vi "Status Monitor (Multi Unit).vi"() -> ()   [LabVIEW 2017, in "Status Monitor Library.lvlib"]
uses:
  Status Monitor Library.lvlib
  Communications/Typedefs/DTACQ Module Carrier Status.ctl
  Communications/Typedefs/DTACQ Status--Enum.ctl
  Communications/Communications Library.lvlib
panel:
  in  "error out":errorcluster
  out "Array":T1[](array[typedef])
  in  "stop":bool
  in  "appended array":path[](array[path])
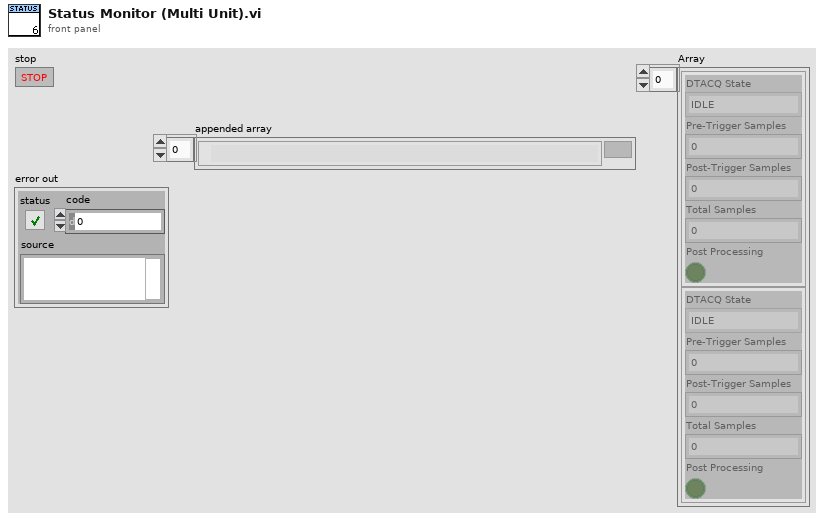
[diagram p1: front panel]
types:
  T1 = typedef "Communications Library.lvlib/DTACQ Module Carrier Status.ctl" = cluster{"DTACQ State":T2, "Pre-Trigger Samples":i32, "Post-Trigger Samples":i32, "Total Samples":i32, "Post Processing":bool}
  T2 = typedef "Communications Library.lvlib/DTACQ Status--Enum.ctl" = enum16{"IDLE", "ARM", "RUN_PRE-TRIGGER", "RUN_POST-TRIGGER", "POST_PROCESS", "CLEANUP"}
  T3 = typedef "Communications Library.lvlib/DTACQ Connection Data--Cluster.ctl" = cluster{"Description":string, "Address":string, "Port":u16, "timeout (ms)":i32, "Termination Character":string, "TCP Connection Reference":refnum<k5>, "Open Connection":bool}
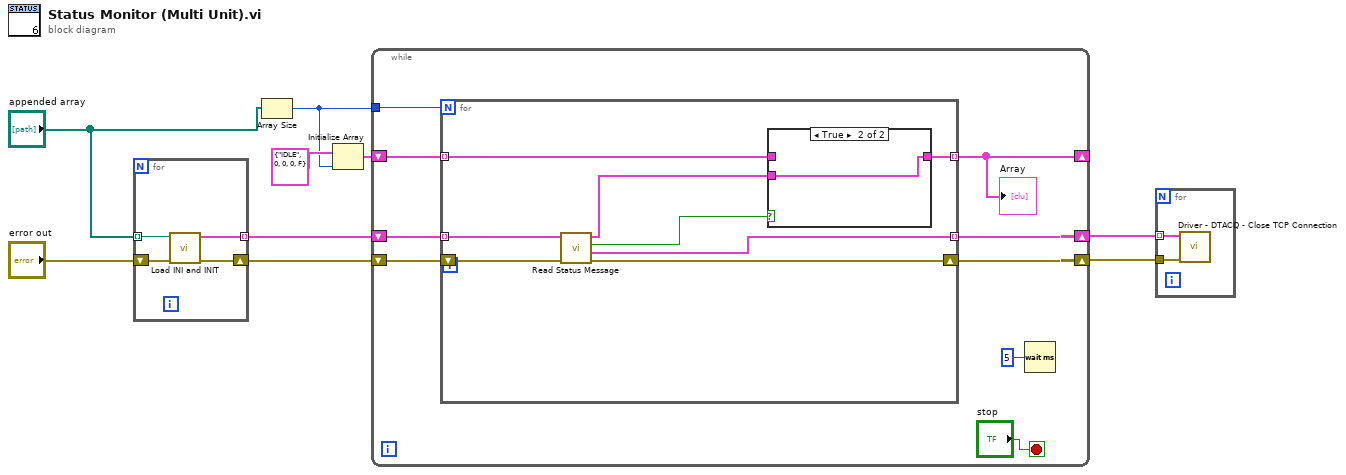
[diagram p0: block diagram]
diagram:
  n1 = for {
    tunnel: "appended array" -> [w13] mode=indexing
    shift-right: [w12] -> w9
    shift-left: "error out" -> [w11]
    tunnel: [w10] -> w1 mode=indexing
    n2 = call "Load INI and INIT.vi"("error in (no error)"=w11, "configuration file path"=w13) -> ("error out"=w12:errorcluster, "Status Connection Out"=w10:T3)  [unwired: 8 in]
  }
  n3 = Array Size(array="appended array") -> (size(s)=w3:i32)
  n4 = Initialize Array(T1 {"DTACQ State"=enum."IDLE", "Pre-Trigger Samples"=0, "Post-Trigger Samples"=0, "Total Samples"=0, "Post Processing"=FALSE} ("Module Carrier Status"), w3) -> (w5:T1[])
  n5 = while {
    shift-right: [w20] -> w8
    shift-left: w1 -> [w16]
    shift-right: [w21] -> w7
    shift-left: w9 -> [w22]
    shift-right: [w18] -> _
    shift-left: w5 -> [w17]
    tunnel: w3 -> [w14]
    stop <- "stop" stop-if-true
    n6 = for {
      N: w14 -> [_]
      tunnel: w16 -> [w30] mode=indexing
      shift-right: [w27] -> w21
      shift-left: w22 -> [w29]
      tunnel: [w28] -> w20 mode=indexing
      tunnel: [w23] -> w18 mode=indexing
      tunnel: w17 -> [w24] mode=indexing
      n7 = call "Read Status Message.vi"("error in (no error)"=w29, "Status Connection Out"=w30) -> ("error out"=w27:errorcluster, "DTACQ Connection Data Out"=w28:T3, "New Status Message"=w26:bool, "Module Carrier Status"=w25:T1)  [unwired: 6 in]
      n8 = case shown="True" w26 {
        tunnel: w25 -> [_ w32]
        tunnel: [w31 w32] -> w23
        tunnel: w24 -> [w31 _]
        frame False {
        }
        frame True {
        }
      }
    }
    "Array" <- w18
    n9 = Wait (ms)(milliseconds to wait=u32 5) -> ()  [unwired: 1 out]
  }
  n10 = for {
    tunnel: w8 -> [w34] mode=indexing
    tunnel: w7 -> [w33]
    n11 = call "Driver - DTACQ - Close TCP Connection.vi"("error in"=w33, "DTACQ Connection Data In"=w34) -> ()  [unwired: 8 in, 2 out]
  }
